vi "Linhas XY-trigger.vi"() -> ()   [LabVIEW 2014]
doc: "André Romero - 2023\nandretec@ifsc.usp.br\nIFSC - USP"
panel:
  out "Boolean":bool
  in  "stop":bool
  out "Progress":i32=56
  out "Stop":bool
  in  "Acc":dbl=0.45
  in  "Velocity":sgl=0.45
  out "Motor M1":bool=TRUE
  out "Motor M2":bool=TRUE
  in  "Swap motor":bool
  in  "d (um)":dbl=1.0
  in  "L (um)":dbl=500.0
  in  "N Lines":i32=100
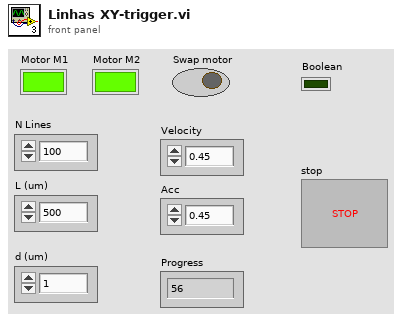
[diagram p1: front panel]
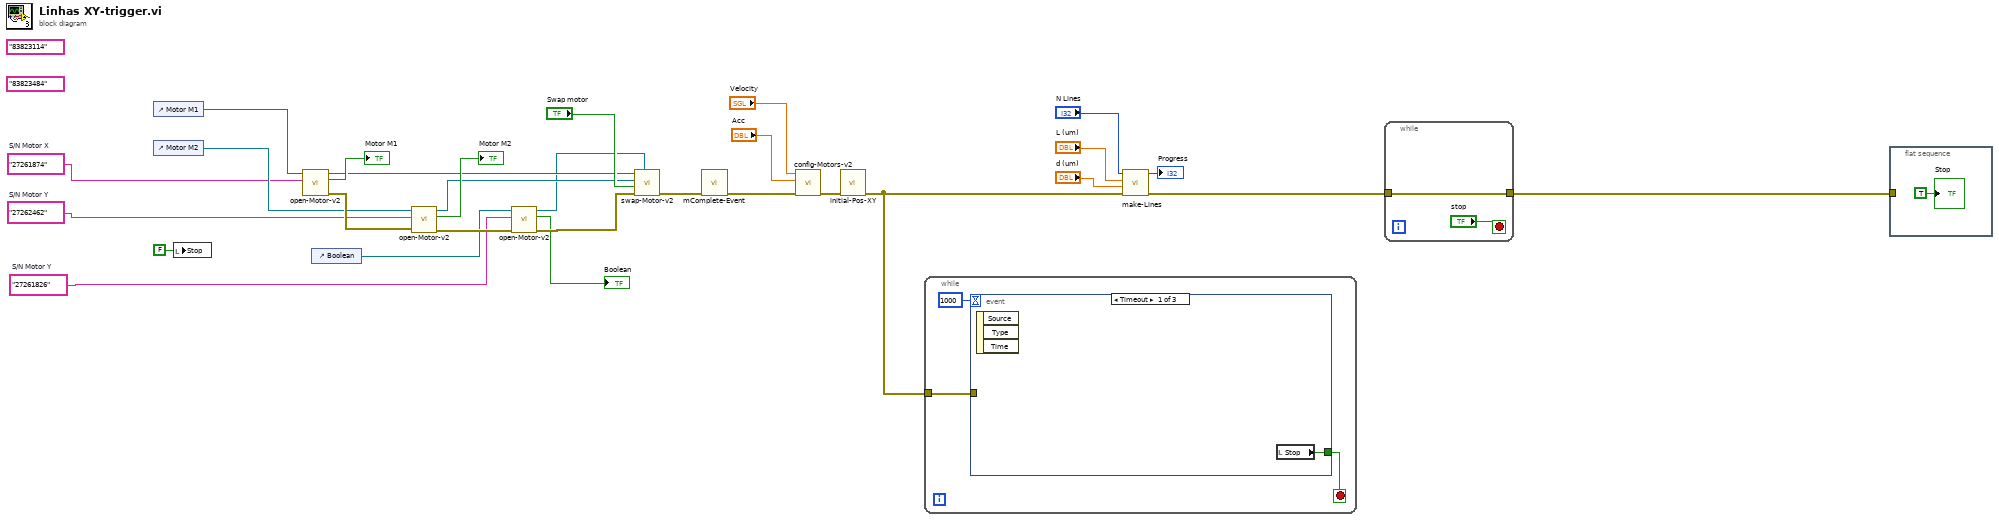
[diagram p0: block diagram]
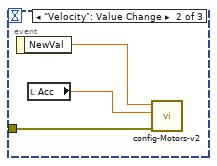
[diagram p2: hidden frame]
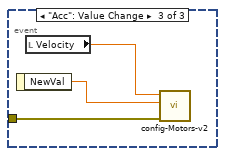
[diagram p3: hidden frame]
diagram:
  w7 = "27261826"  # S/N Motor Y
  w10 = "27262462"  # S/N Motor Y
  w11 = "27261874"  # S/N Motor X
  (unwired) "83823484" ("S/N Motor")
  (unwired) "83823114" ("S/N Motor")
  n1 = control-ref of="Motor M1"() -> (w25:refnum<vi>)
  n2 = control-ref of="Motor M2"() -> (w24:refnum<vi>)
  n3 = local write "Stop"(FALSE ("Stop")) -> ()
  n4 = call "open-Motor-v2.vi"("S/N Motor"=w11, "ref Boolean in"=w25) -> ("Error Out"=w29:errorcluster, "Motor Status"=→"Motor M1":bool, "Refnum out"=w13:refnum<k7>)  [unwired: 7 in]
  n5 = control-ref of="Boolean"() -> (w4:refnum<vi>)
  n6 = call "open-Motor-v2.vi"("Error In"=w29, "S/N Motor"=w10, "ref Boolean in"=w24) -> ("Error Out"=w9:errorcluster, "Motor Status"=→"Motor M2":bool, "Refnum out"=w12:refnum<k7>)  [unwired: 6 in]
  n7 = call "open-Motor-v2.vi"("Error In"=w9, "S/N Motor"=w7, "ref Boolean in"=w4) -> ("Error Out"=w8:errorcluster, "Motor Status"=→"Boolean":bool, "Refnum out"=w6:refnum<k7>)  [unwired: 6 in]
  n8 = call "swap-Motor-v2.vi"("Refnum in M3"=w6, "error in (no error)"=w8, "Swap motor"="Swap motor", "Refnum in M2"=w12, "Refnum in M1"=w13) -> ("error out"=w2:errorcluster)  [unwired: 6 in]
  n9 = call "mComplete-Event.vi"("Error In"=w2) -> ("Error Out"=w1:errorcluster)  [unwired: 10 in]
  n10 = call "config-Motors-v2.vi"("error in"=w1, "Acc"="Acc", "Velocity"="Velocity") -> ("error out"=w17:errorcluster)  [unwired: 8 in]
  n11 = call "initial-Pos-XY.vi"("error in (no error)"=w17) -> ("error out"=w16:errorcluster)  [unwired: 8 in, 2 out]
  n12 = while {
    tunnel: w16 -> [w30]
    stop <- w31 stop-if-true
    n13 = event shown="[0] Timeout" {
      selector: _ -> [_ _ _]
      dyn-events: _ -> [_ _ _]
      timeout: 1000 -> [_ _ _]
      tunnel: [w33 _ _] -> w31
      tunnel: w30 -> [_ w36 w39]
      event Timeout {
        n14 = event-data() -> ()  [unwired: 1 in, 3 out]
        n15 = local read "Stop"() -> (w33:bool)
      }
      event "Velocity": Value Change {
        n16 = event-data() -> ("NewVal"=w35:sgl)  [unwired: 1 in]
        n17 = local read "Acc"() -> (w34:dbl)
        n18 = call "config-Motors-v2.vi"("error in"=w36, "Acc"=w34, "Velocity"=w35) -> ()  [unwired: 8 in, 1 out]
      }
      event "Acc": Value Change {
        n19 = event-data() -> ("NewVal"=w37:dbl)  [unwired: 1 in]
        n20 = local read "Velocity"() -> (w38:sgl)
        n21 = call "config-Motors-v2.vi"("error in"=w39, "Acc"=w37, "Velocity"=w38) -> ()  [unwired: 8 in, 1 out]
      }
    }
  }
  n22 = call "make-Lines.vi"("error in"=w16, "d (um)"="d (um)", "L (um)"="L (um)", "N Lines"="N Lines") -> ("error out"=w15:errorcluster, "Progress"=→"Progress":i32)  [unwired: 6 in]
  n23 = while {
    tunnel: w15 -> [w40]
    tunnel: [w40] -> w3
    stop <- "stop" stop-if-true
  }
  n24 = flat-sequence {
    tunnel: w3 -> [_]
    frame #0 {
      "Stop" <- TRUE ("Stop")
    }
  }
